vi "Hyphenation.vi"(8 "error in":errorcluster, 11 "Word":string) -> (0 "error out":errorcluster, 3 "Hyphenated":string[](array[string]))   [LabVIEW 2020, in "Silly Billy.lvlib"]
doc: "Odd numbers indicate that hyphenation is allowed at that index"
uses:
  Silly Billy.lvlib
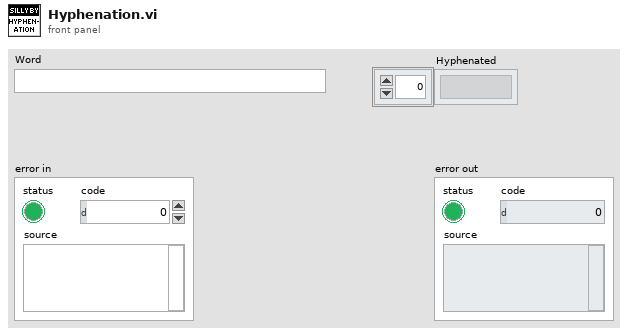
[diagram p1: front panel]
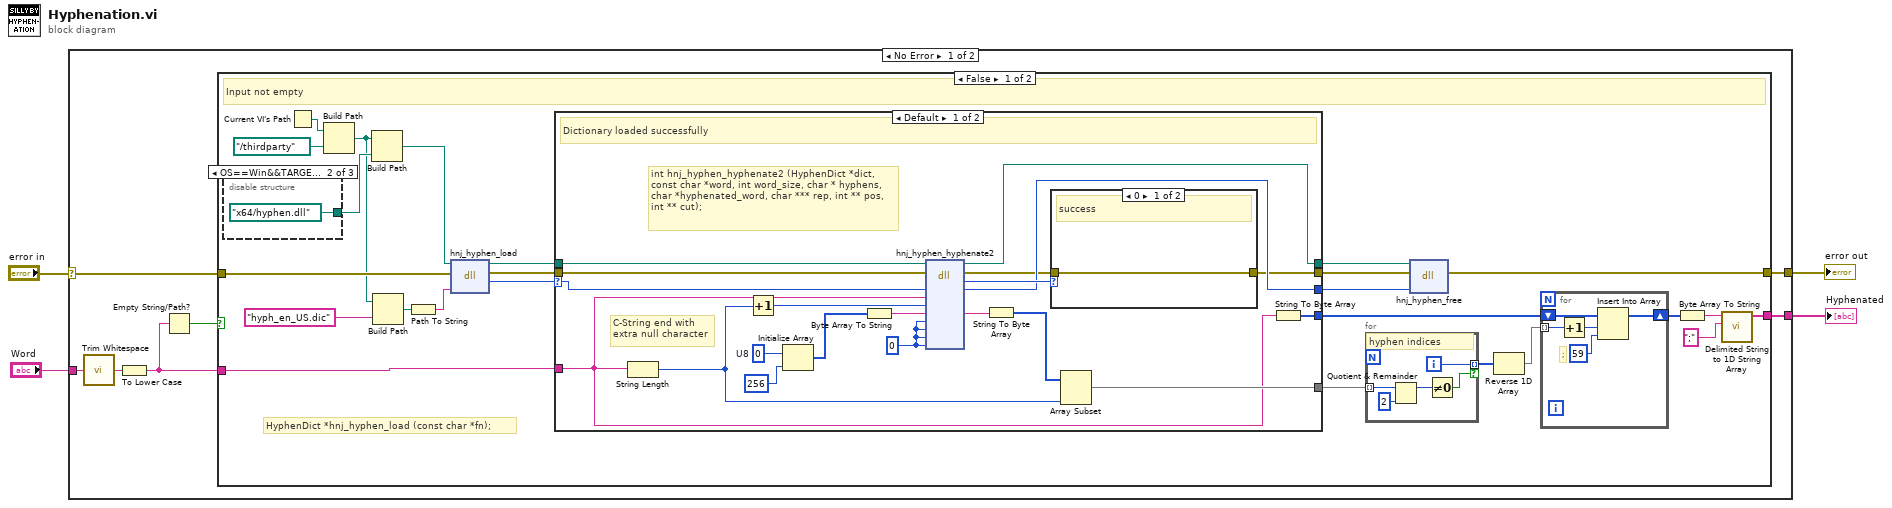
[diagram p0: block diagram]
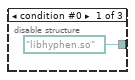
[diagram p2: hidden frame]
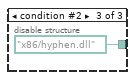
[diagram p3: hidden frame]
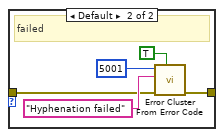
[diagram p4: hidden frame]
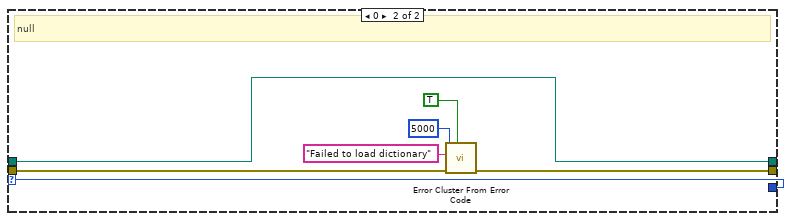
[diagram p5: hidden frame]
diagram:
  n1 = case shown="No Error" "error in" {
    selector: "error in" -> [w11 w84]
    tunnel: [w10 w84] -> w3
    tunnel: "Word" -> [w9 _]
    tunnel: [w5 _] -> w1
    frame No Error {
      n2 = call <vilib>:"Trim Whitespace.vi"("string"=w9) -> ("trimmed string"=w7:string)  [unwired: 1 in]
      n3 = To Lower Case(string=w7) -> (all lower case string=w6:string)
      n4 = Empty String/Path?(string/path=w6) -> (empty?=w8:bool)
      n5 = case shown="False" w8 {
        tunnel: w11 -> [w36 w83]
        tunnel: [w32 w83] -> w10
        tunnel: w6 -> [w30 _]
        tunnel: [w14 _] -> w5
        frame False {
          # "HyphenDict *hnj_hyphen_load (const char *fn);"
          # "Input not empty"
          n6 = disable-structure shown="OS==Win&&TARGET_BITNESS==64, Default" {
            disable-tunnel: [path "libhyphen.so" ("path in") path "x64/hyphen.dll" ("path in") path "x86/hyphen.dll" ("path in")] -> w25
            frame condition #0 {
            }
            frame condition #1 (active) {
            }
            frame condition #2 {
            }
          }
          n7 = Current VI's Path() -> (path=w27:path)
          n8 = Build Path(base path=w27, name or relative path=path "../thirdparty") -> (appended path=w23:path)
          n9 = Build Path(base path=w23, name or relative path=w25) -> (appended path=w24:path)
          n10 = Build Path(base path=w23, name or relative path="hyph_en_US.dic") -> (appended path=w21:path)
          n11 = Path To String(path=w21) -> (string=w20:string)
          n12 = dll-call lib="?" fn="hnj_hyphen_load"(path in=w24, error in=w36, ".dic"=w20) -> (path out=w31:path, error out=w35:errorcluster, "return type"=w34:u64)  [unwired: 2 in]
          n13 = case shown="Default" w34 {
            selector: w34 -> [w67 w76]
            tunnel: w35 -> [w69 w82]
            tunnel: [w62 w81] -> w33
            tunnel: w31 -> [w68 w77]
            tunnel: w30 -> [w51 _]
            tunnel: [w65 w76] -> w29
            tunnel: [w64 w77] -> w28
            tunnel: [w52 _] -> w19
            tunnel: [w50 _] -> w13
            frame Default {
              w59 = u64 0
              w60 = u8 0  # U8
              # "C-String end with\nextra null character"
              # "int hnj_hyphen_hyphenate2 (HyphenDict *dict, const char *word, int word_size, char * hyphens, char *hyphenated_word, char *** rep, int ** pos, int ** cut);"
              # "Dictionary loaded successfully"
              n14 = String Length(string=w51) -> (length=w53:i32)
              n15 = Increment(x=w53) -> (x+1=w57:i32)
              n16 = Initialize Array(w60, 256 ("y")) -> (w61:u8[])
              n17 = Byte Array To String(unsigned byte array=w61) -> (string=w58:string)
              n18 = dll-call lib="?" fn="hnj_hyphen_hyphenate2"(path in=w68, error in=w69, "dict"=w67, "word"=w51, "word_size"=w57, "hyphens"=w58, "hyphenated_word"=w59, "rep"=w59, "pos"=w59, "cut"=w59) -> (path out=w64:path, error out=w63:errorcluster, "return type"=w66:i32, "dict"=w65:u64, "hyphens"=w55:string)  [unwired: 7 in]
              n19 = String To Byte Array(string=w55) -> (unsigned byte array=w54:u8[])
              n20 = case shown="0" w66 {
                tunnel: w63 -> [w70 w73]
                tunnel: [w70 w72] -> w62
                frame 0 {
                  # "success"
                }
                frame Default {
                  # "failed"
                  n21 = call <vilib>:"Error Cluster From Error Code.vi"("show call chain? (False)"=TRUE, "error in (no error)"=w73, "error message (\"\")"="Hyphenation failed" ("error message (\"\")"), "error code (0)"=5001) -> ("error out"=w72:errorcluster)  [unwired: 5 in]
                }
              }
              n22 = Array Subset(array=w54, length=w53) -> (w52:u8[])  [unwired: 1 in]
              n23 = String To Byte Array(string=w51) -> (unsigned byte array=w50:u8[])
            }
            frame 0 {
              # "null"
              n24 = call <vilib>:"Error Cluster From Error Code.vi"("show call chain? (False)"=TRUE, "error in (no error)"=w82, "error message (\"\")"="Failed to load dictionary" ("error message (\"\")"), "error code (0)"=5000) -> ("error out"=w81:errorcluster)  [unwired: 5 in]
            }
          }
          n25 = for {
            tunnel: w19 -> [w46] mode=indexing
            tunnel: [w43] -> w18 mode=indexing if=w42
            i -> [w43]
            # "hyphen indices"
            n26 = Quotient & Remainder(x=w46, y=2) -> (x-y*floor(x/y)=w44:i32)  [unwired: 1 out]
            n27 = Not Equal To 0?(x=w44) -> (x != 0?=w42:bool)
          }
          n28 = dll-call lib="?" fn="hnj_hyphen_free"(path in=w28, error in=w33, "dic"=w29) -> (error out=w32:errorcluster)  [unwired: 3 in, 1 out]
          n29 = Reverse 1D Array(array=w18) -> (reversed array=w12:i32[])
          n30 = for {
            shift-right: [w39] -> w17
            shift-left: w13 -> [w41]
            tunnel: w12 -> [w38] mode=indexing
            # ";"
            n31 = Increment(x=w38) -> (x+1=w37:i32)
            n32 = Insert Into Array(array=w41, index=w37, new element=u8 59 ("new element/subarray")) -> (w39:u8[])
          }
          n33 = Byte Array To String(unsigned byte array=w17) -> (string=w16:string)
          n34 = call <vilib>:"Delimited String to 1D String Array.vi"("delimiter"=";", "delimited string"=w16) -> ("string array"=w14:string[])  [unwired: 9 in]
        }
        frame True {
          # "Input empty"
        }
      }
    }
    frame Error {
    }
  }
  "error out" <- w3
  "Hyphenated" <- w1
